vi "SubscriberExample.vi"() -> ()   [LabVIEW 2015]
doc: "Sample subscriber. Subscribes to the topic chatter"
uses:
  ROS/Code/Console/Servers/ServerSubs/TopicDef.ctl
  ROS/Code/SubVIs/_ROSDirection.ctl
  ROS/MessageParsing/std_msgs/subs/parse_string_scalar.vi
panel:
  in  "stop":bool
  out "error out":errorcluster
  out "I heard:":string
  # "Instructions:\n1. Run Publisher example\n2. Run Subscriber eample"
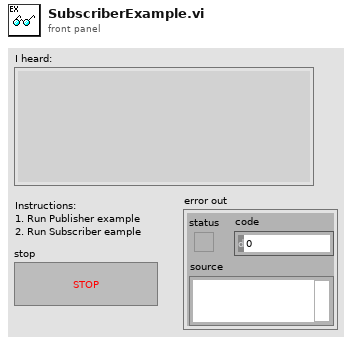
[diagram p1: front panel]
types:
  T1 = typedef "TopicDef.ctl" = cluster{"Topic":string, "Type":string, "Action":T2, "Update (ms)":u16, "queue size":u16}
  T2 = typedef "_ROSDirection.ctl" = enum16{"Node", "Publisher", "Subscriber", "ServiceClient", "ServiceProvider"}
  T3 = typedef "_ROSControl.ctl" = cluster{"topic port":u16, "Node":string, "topic":string, "type":string, "node port":u16, "error ":errorcluster, "Direction":T2, "Update (ms)":u16, "FIFO size":u16}
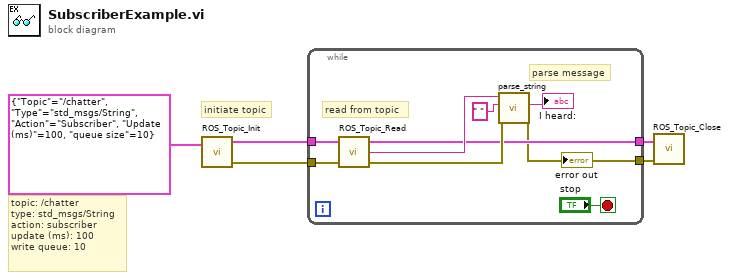
[diagram p0: block diagram]
diagram:
  # "initiate topic"
  # "topic: /chatter\ntype: std_msgs/String\naction: subscriber\nupdate (ms): 100\nwrite queue: 10"
  n1 = call "ROS_Topic_Init.vi"("Definitions"=T1 {"Topic"="/chatter", "Type"="std_msgs/String", "Action"=enum."Subscriber", "Update (ms)"=100, "queue size"=10}) -> ("ROS out"=w4:T3, "error out"=w3:errorcluster)  [unwired: 2 in]
  n2 = while {
    tunnel: w4 -> [w14]
    tunnel: w3 -> [w10]
    tunnel: [w7] -> w2
    tunnel: [w6] -> w1
    stop <- "stop" stop-if-true
    # "parse message"
    # "read from topic"
    n3 = call "ROS_Topic_Read.vi"("error in (no error)"=w10, "ROS in"=w14) -> ("error out"=w9:errorcluster, "Reply"=w13:string, "ROS out"=w7:T3)  [unwired: 1 in]
    n4 = call-poly "parse_string.vi"("error in"=w9, "type"=" ", "msg in"=w13) -> ("error out"=w6:errorcluster, "string"=→"I heard:":string)  [unwired: 2 in, 1 out]
    "error out" <- w6
  }
  n5 = call "ROS_Topic_Close.vi"("error in"=w1, "ROS in"=w2) -> ()  [unwired: 2 in, 1 out]
